vi "Pre Launch Init.vi"(11 "State Machine Actor in":refnum<class "State Machine Actor.lvclass">) -> (0 "error out":errorcluster, 3 "State Machine Actor out":refnum<class "State Machine Actor.lvclass">)   [LabVIEW 2024, in "State Machine Actor.lvlib" / "State Machine Actor.lvclass"]
doc: "<p>(<strong>Filename</strong>: <span class=\"dnl\">Actor Framework.lvlib:Actor.lvclass:Pre Launch Init.vi</span>)</p>\n<p>Defines behavior that occurs after the <a href=\"nihelplauncher://docs/csh?context=lvcore_lvcomm_af_launch_nested_actor\">Launch Nested Actor</a> method is invoked but before the actor's Actor Core method begins running.</p>\n<p>By default, this method does nothing. A descendant class may override it to define behavior.</p>"
uses:
  State Machine Actor.lvclass
  State Machine Actor.lvclass/State Machine Actor.ctl
  _State Machine Actor/_State Machine Actor/_State Machine Actor.lvclass
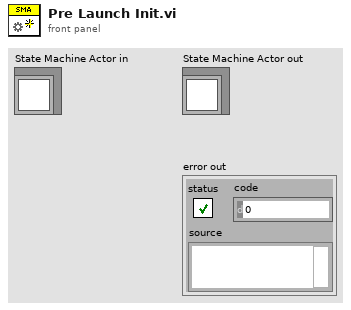
[diagram p1: front panel]
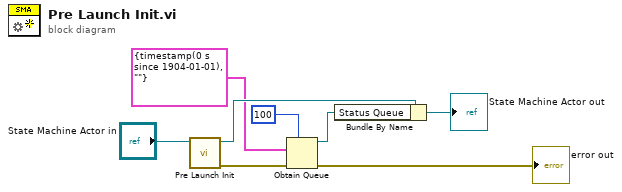
[diagram p0: block diagram]
diagram:
  n1 = call-parent "Pre Launch Init.vi"("Actor in"="State Machine Actor in") -> ("error out"=w4:errorcluster, "Actor out"=w7:refnum<class "State Machine Actor.lvclass">)  [unwired: 9 in]
  n2 = Obtain Queue(max queue size (-1, unlimited)=100, element data type=cluster{timestamp, string} {timestamp(0 s since 1904-01-01), ""}, error in (no error)=w4) -> (queue out=w2:refnum<queue>, error out=→"error out":errorcluster)  [unwired: 2 in, 1 out]
  n3 = Bundle By Name(cluster=w7, "Status Queue"=w2) -> (→"State Machine Actor out":refnum<class "State Machine Actor.lvclass">)
